vi "Stop Core.vi"(10 "final error code":i32, 11 "Freezer in":refnum<class "Freezer.lvclass">) -> (3 "Freezer out":refnum<class "Freezer.lvclass">)   [LabVIEW 2015, in "cRIO-Carbondioxide.lvlib" / "CO2-Actor.lvlib" / "Freezer.lvclass"]
doc: "(<B>Filename</B>: Actor Framework.lvlib:Actor.lvclass:Stop Core.vi)\n\nDefines what the actor does before it stops. Use the <B>final error code</B> input to determine whether the actor shut down in response to an error.\n\nBy default, this method does nothing. A descendant class may override it to define behavior, such as shutting down any processes the actor initiated in its override of the Actor Core method."
uses:
  Freezer.lvclass
  Freezer.lvclass/Freezer.ctl
  CO2 Actor/CO2 Actor.lvclass
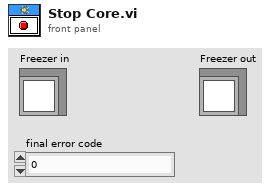
[diagram p1: front panel]
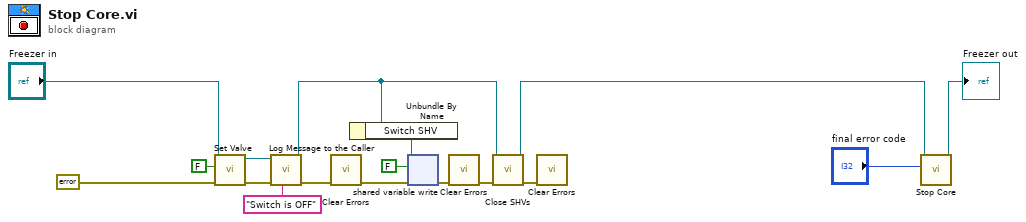
[diagram p0: block diagram]
diagram:
  n1 = call "Set Valve.vi"("error in (no error)"=errorcluster {"status"=FALSE, "code"=0, "source"=""}, "Open/Close"=FALSE, "Freezer in"="Freezer in") -> ("error out"=w8:errorcluster, "Freezer out"=w6:refnum<class "Freezer.lvclass">)  [unwired: 7 in]
  n2 = call-dynamic "Log Message to the Caller.vi"("String (\"\" = no message to send)"="Switch is OFF" ("String"), "error in (no error)"=w8, "CO2 Actor in"=w6) -> ("error out"=w7:errorcluster, "CO2 Actor out"=w5:refnum<class "Freezer.lvclass">)  [unwired: 7 in]
  n3 = call <vilib>:"Clear Errors.vi"("error in (no error)"=w7) -> ("error out"=w13:errorcluster)  [unwired: 5 in, 1 out]
  n4 = Unbundle By Name(w5) -> ("Switch SHV"=w12:refnum<k21>)
  n5 = shared-variable-write(w12, w13, FALSE ("data in")) -> (w11:errorcluster)  [unwired: 1 out]
  n6 = call <vilib>:"Clear Errors.vi"("error in (no error)"=w11) -> ("error out"=w10:errorcluster)  [unwired: 5 in, 1 out]
  n7 = call "Close SHVs.vi"("error in (no error)"=w10, "Freezer in"=w5) -> ("error out"=w2:errorcluster, "Freezer out"=w1:refnum<class "Freezer.lvclass">)  [unwired: 8 in]
  n8 = call <vilib>:"Clear Errors.vi"("error in (no error)"=w2) -> ()  [unwired: 5 in, 2 out]
  n9 = call-parent "Stop Core.vi"("final error code"="final error code", "CO2 Actor in"=w1) -> ("CO2 Actor out"=→"Freezer out":refnum<class "Freezer.lvclass">)  [unwired: 9 in]
